vi "Example_OE1311&1351 Control.vi"() -> ()   [LabVIEW 2011]
uses:
  <vilib>/Utility/error.llb/DialogType.ctl
panel:
  out "loss count":i32=-1
  in  "Sample count":u32
  in  "buffer":u8
  out "Zero Data?":bool
  out "Queue out":errorcluster caption="error out"
  out "Queue output":refnum<queue>
  in  "Timeout":u32=100
  in  "Port":u32=10001
  in  "IP Address":string
  out "Freq":dbl
  out "xita":dbl
  out "R":dbl
  out "Input Overlaod":bool
  out "PLL Lock":bool
  out "Error":string
  out "Serial Versions":string
  in  "Table":T1(tab) caption="选项卡控件"
  in  "OE1300_Configure Input Filter":T2 {"Input Coupling" items=["AC", "DC"]; "Input Source" items=["A", "B", "Current"]}
  in  "OE1300_Configure Ref Phase":T3={"Reference Source"=0, "Internal Frequency(Hz)"=1000.0, "Phase  (degree)"=0.0, "External Ref Trigger"=0, "Instrument Mode "=4} {"Instrument Mode" items=["OE1311"=3, "OE1351"=4, "OE1301"=5]; "External Ref Trigger" items=["TTL Rising Edge", "TTL Fallling Edge", "Sine Zero Crossing"]; "Phase  (degree)" min=-180.0 max=180.0 format="%#.2g"; "Internal Frequency(Hz)" min=0.001 max=1002000.0 format="%#.3f"; "Reference Source" items=["External", "Internal", "Self"]}
  in  "OE1300_Configure Sens and Filter":T4={"Time Constant(s) "=0.1, "Low Pass Filter Slope "=1, "Enable Sync Filter "=0, "Input Range"=2} {"Input Range" items=["5 V/uA", "2 V/uA", "1 V/uA", "500 mV/nA", "200 mV/nA", "100 mV/nA", "50 mV/nA", "20 mV/nA", "10 mV/nA", "5 mV/nA", "2 mV/nA", "1 mV/nA", "500 uV/pA", "200 uV/pA", "100 uV/pA", "50 uV/pA", "20 uV/pA", "10 uV/pA", "5 uV/pA", "2 uV/pA", "1 uV/pA", "500 nV/fA", "200 nV/fA", "100 nV/fA", "50 nV/fA", "20 nV/fA", "10 nV/fA", "5 nV/fA", "2 nV/fA", "1 nV/fA"]; "Enable Sync Filter" items=["OFF", "ON"]; "Low Pass Filter Slope" items=["6 dB/oct", "12 dB/oct", "18 db/oct", "24 dB/oct", "30 dB/oct", "36 dB/oct", "42 dB/oct", "48 dB/oct"]; "Time Constant(s)" min=1e-06 max=3000.0}
  in  "OE1300_Configure Channel Out":T5={"CH2 Offset"=0.0, "CH1 Offset"=0.0, "CH2 Expand"=1, "CH1 Expand"=1, "AUX OUT1"=1.0, "AUX OUT2"=1.0, "CH 1"=3, "CH 2"=3} {"CH 2" items=["Fixed", "X", "Y", "R", "Theta", "Xh1", "Yh1", "Rh1", "Theta h1", "Xh2", "Yh2", "Rh2", "Theta h2", "Xh3", "Yh3", "Rh3", "Theta h3", "Rh4", "Xh4", "Yh4", "Theta h4", "Rh5", "Xh5", "Yh5", "Theta h5", "Rh6", "Xh6", "Yh6", "Theta h6", "Rh7", "Xh6", "Yh6", "Theta h7", "X_Noise", "Y_Noise", "Freq", "AuxIn1", "AuxIn2"]; "CH 1" items=["Fixed", "X", "Y", "R", "Theta", "Xh1", "Yh1", "Rh1", "Theta h1", "Xh2", "Yh2", "Rh2", "Theta h2", "Xh3", "Yh3", "Rh3", "Theta h3", "Rh4", "Xh4", "Yh4", "Theta h4", "Rh5", "Xh5", "Yh5", "Theta h5", "Rh6", "Xh6", "Yh6", "Theta h6", "Rh7", "Xh6", "Yh6", "Theta h7", "X_Noise", "Y_Noise", "Freq", "AuxIn1", "AuxIn2"]; "AUX OUT2" min=-10.0 max=10.0 format="%#.3g"; "AUX OUT1" min=-10.0 max=10.0 format="%#.3g"; "CH1 Expand" min=1 max=256; "CH2 Expand" min=1 max=256; "CH1 Offset" min=-100.0 max=100.0 format="%#.2g"; "CH2 Offset" min=-100.0 max=100.0 format="%#.2g"}
  in  "OE1300_Configure Sine Out":T6={"Sine Output Amplitude (V)"=0.1, "SineOut Mode"=0} {"SineOut Mode" items=["OFF", "Fixed"]; "Sine Output Amplitude (V)" min=0.0001 max=5.0 format="%#.4g"}
  in  "OE1300_Configure Demodulator":T7={"Demodulator"=1, "Mode"=0, "Arbitrary Frequency"=1000.0, "Harmonic"=1, "Instrument Mode "=4, "Phase  (degree)"=0.0} {"Phase  (degree)" min=-180.0 max=180.0 format="%#.2g"; "Instrument Mode" items=["OE1311"=3, "OE1351"=4, "OE1301"=5]; "Harmonic" min=1 max=32767; "Arbitrary Frequency" min=1e-06 max=1002000.0 format="%#.3f"; "Mode" items=["Harm", "Arb_Freq"]; "Demodulator" items=["1", "2", "3", "4", "5", "6", "7"]}
  in  "Save Button":bool
  in  "file path":path
  in  "Sample Rate":dbl=0.1 min=0.001 max=100.0
  out "Status":string
  in  "Connect":bool
  in  "VISA resource name":refnum<visa-resource-name>
  in  "Remote Mode":u16(ring)=1 items=["RS232"=1, "Ethernet"=3]
  in  "Baud Rate (115200)":u32=115200
  # "Tel          :   +86-020-84133345\nWebsite  :   www.ssi-instrument.com\nE-mail     :   support@si-instrument.com"
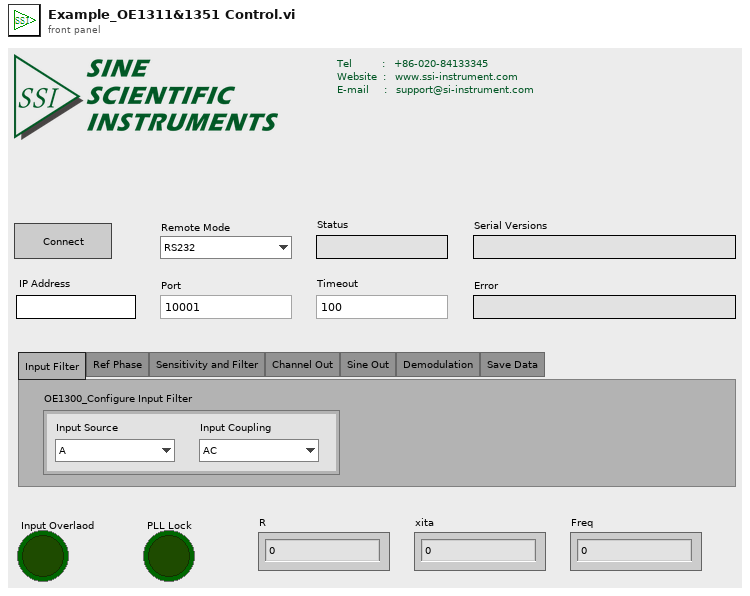
[diagram p1: front panel]
types:
  T1 = enum32{"Input Filter", "Ref Phase", "Sensitivity and Filter", "Channel Out", "Sine Out", "Demodulation", "Save Data"}
  T2 = cluster{"Input Source":u16, "Input Coupling ":u16}
  T3 = cluster{"Reference Source":u16, "Internal Frequency(Hz)":dbl, "Phase  (degree)":dbl, "External Ref Trigger":u16, "Instrument Mode ":u16}
  T4 = cluster{"Time Constant(s) ":dbl, "Low Pass Filter Slope ":u8, "Enable Sync Filter ":u16, "Input Range":u16}
  T5 = cluster{"CH2 Offset":dbl, "CH1 Offset":dbl, "CH2 Expand":i16, "CH1 Expand":i16, "AUX OUT1":dbl, "AUX OUT2":dbl, "CH 1":u16, "CH 2":u16}
  T6 = cluster{"Sine Output Amplitude (V)":dbl, "SineOut Mode":u8}
  T7 = cluster{"Demodulator":u16, "Mode":u16, "Arbitrary Frequency":dbl, "Harmonic":u16, "Instrument Mode ":u16, "Phase  (degree)":dbl}
  T8 = enum16{"OE1022", "OE1022D", "OE1201", "OE2031&OE2041", "OE1311&OE1351"}
  T9 = cluster{"Port":u32, "Timeout":u32, "IP Address":string}
  T10 = cluster{"PLL Lock(1: External Lock)":bool, "Input Overlaod":bool}
  T11 = cluster{"X":dbl, "Y":dbl, "R":dbl, "θ":dbl, "XD1":dbl, "YD1":dbl, "RD1":dbl, "θD1":dbl, "XD2":dbl, "YD2":dbl, "RD2":dbl, "θD2":dbl, "XD3":dbl, "YD3":dbl, "RD3":dbl, "θD3":dbl, "XD4":dbl, "YD4":dbl, "RD4":dbl, "θD4":dbl, "XD5":dbl, "YD5":dbl, "RD5":dbl, "θD5":dbl, "XD6":dbl, "YD6":dbl, "RD6":dbl, "θD6":dbl, "XD7":dbl, "YD7":dbl, "RD7":dbl, "θD7":dbl, "X-Noise":dbl, "Y-Noise":dbl, "Frequency":dbl, "AUX-IN1":dbl, "AUX-IN2":dbl}
  T12 = typedef "DialogType.ctl" = u16
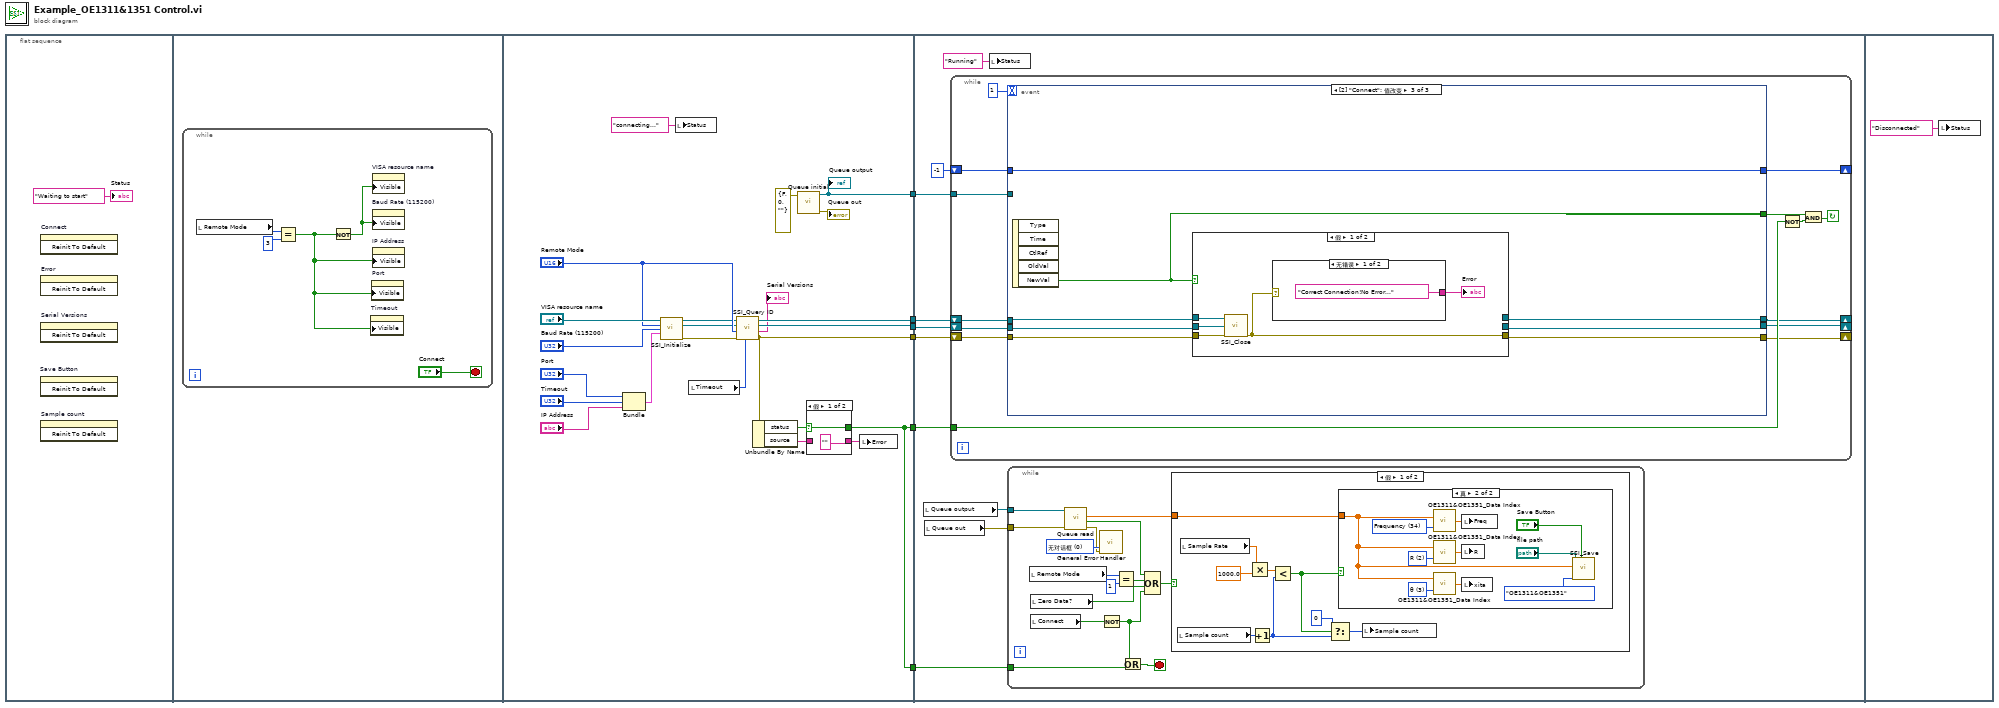
[diagram p0: block diagram]
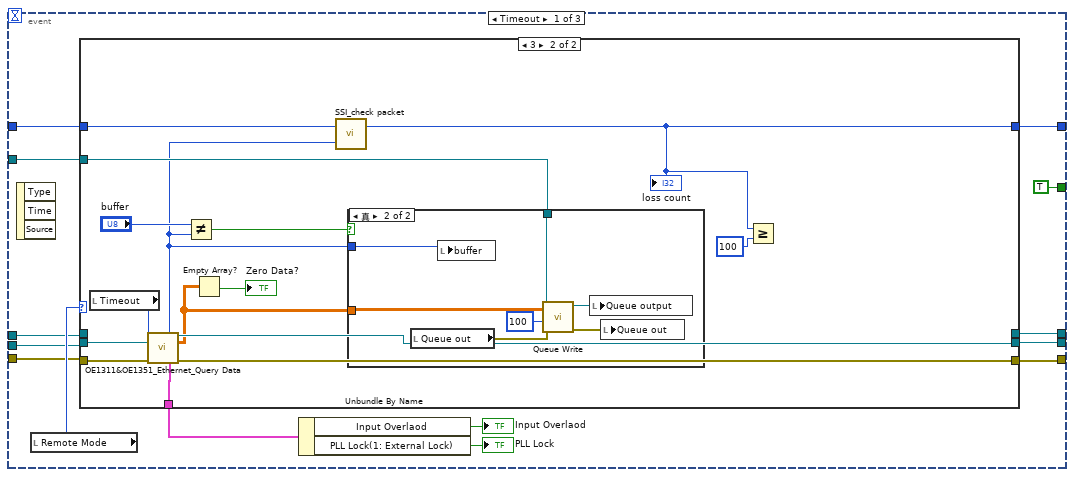
[diagram p5: hidden frame]
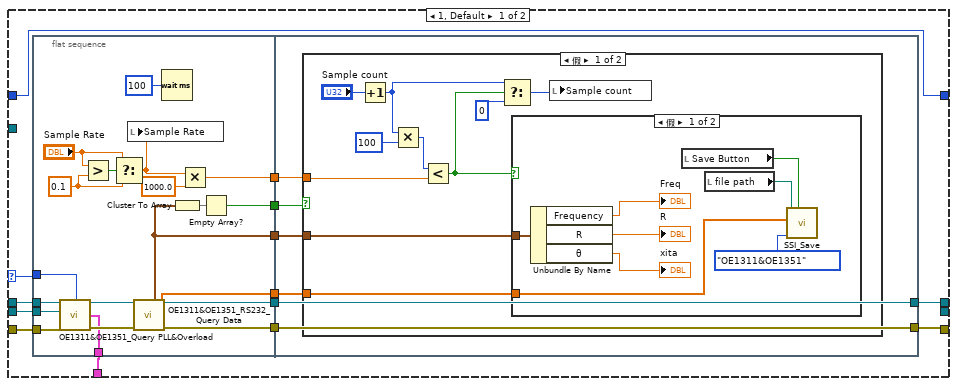
[diagram p6: hidden frame]
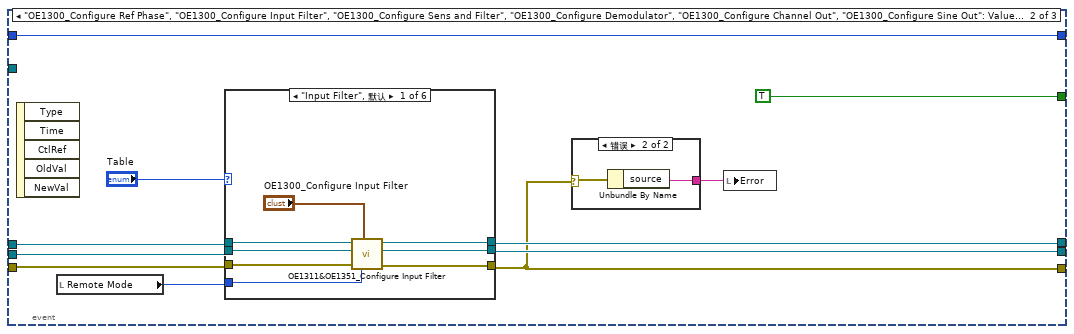
[diagram p10: hidden frame]
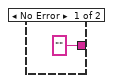
[diagram p11: hidden frame]
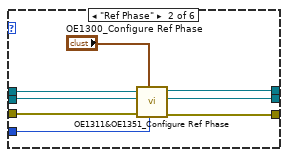
[diagram p12: hidden frame]
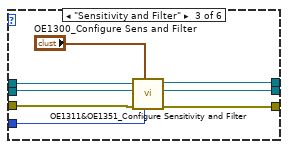
[diagram p13: hidden frame]
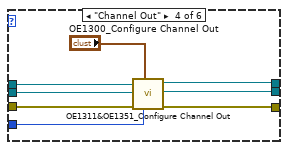
[diagram p14: hidden frame]
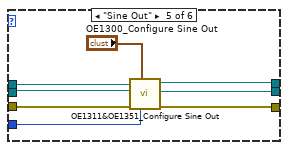
[diagram p15: hidden frame]
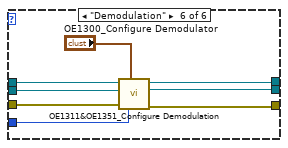
[diagram p16: hidden frame]
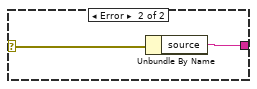
[diagram p17: hidden frame]
diagram:
  n1 = flat-sequence {
    tunnel: [w32] -> w6
    tunnel: [w31] -> w5
    tunnel: [w28] -> w4
    tunnel: [w16] -> w3
    tunnel: [w18] -> w2
    tunnel: [w16] -> w1
    tunnel: w6 -> [w48]
    tunnel: w5 -> [w47]
    tunnel: w4 -> [w46]
    tunnel: w3 -> [w45]
    tunnel: w2 -> [w42]
    tunnel: w1 -> [w40]
    frame #0 {
      n2 = invoke on="Save Button" class="Bool (严格)" method="Reinit To Default"() -> ()  [unwired: 3 in, 3 out]
      n3 = invoke on="Connect" class="Bool (严格)" method="Reinit To Default"() -> ()  [unwired: 3 in, 3 out]
      n4 = invoke on="Error" class="Str" method="Reinit To Default"() -> ()  [unwired: 3 in, 3 out]
      n5 = invoke on="Serial Versions" class="Str" method="Reinit To Default"() -> ()  [unwired: 3 in, 3 out]
      n6 = invoke on="Sample count" class="DigNum (严格)" method="Reinit To Default"() -> ()  [unwired: 3 in, 3 out]
      "Status" <- "Waiting to start" ("status")
    }
    frame #1 {
      n7 = while {
        stop <- "Connect" stop-if-true
        n8 = local read "Remote Mode"() -> (w10:u16)
        n9 = Equal?(x=w10, y=u16 3) -> (x = y?=w11:bool)
        n10 = Not(x=w11) -> (.not. x?=w8:bool)
        n11 = property on="Timeout" class="DigNum (严格)"("Visible"=w11) -> ()  [unwired: 2 in, 2 out]
        n12 = property on="Port" class="DigNum (严格)"("Visible"=w11) -> ()  [unwired: 2 in, 2 out]
        n13 = property on="VISA resource name" class="VISAName"("Visible"=w8) -> ()  [unwired: 2 in, 2 out]
        n14 = property on="Baud Rate (115200)" class="DigNum (严格)"("Visible"=w8) -> ()  [unwired: 2 in, 2 out]
        n15 = property on="IP Address" class="Str"("Visible"=w11) -> ()  [unwired: 2 in, 2 out]
      }
    }
    frame #2 {
      n16 = Bundle("Port"="Port", "Timeout"="Timeout", "IP Address"="IP Address") -> (w23:T9)  [unwired: 1 in]
      n17 = call "SSI_Initialize.vi"("VISA resource name"="VISA resource name", "Remote Mode"="Remote Mode", "baud rate (921600)"="Baud Rate (115200)", "Ethernet"=w23) -> ("VISA resource name out"=w13:refnum<visa-resource-name>, "connection ID(Ethernet)"=w14:refnum<k5>, "error out"=w15:errorcluster)  [unwired: 9 in]
      n18 = local write "Status"("connecting..." ("status")) -> ()
      n19 = local read "Timeout"() -> (w21:u32)
      n20 = call "SSI_Query ID.vi"("Timeout"=w21, "Error in (no error)"=w15, "Remote Mode"="Remote Mode", "Connection ID in"=w14, "VISA resource name"=w13) -> ("Error out"=w28:errorcluster, "Read Buffer"=→"Serial Versions":string, "Connection ID out"=w31:refnum<k5>, "VISA resource  out"=w32:refnum<visa-resource-name>)  [unwired: 3 in]
      n21 = Unbundle By Name(w28) -> ("status"=w29:bool, "source"=w27:string)
      n22 = call "Queue initial.vi"("Error in (no error)"=errorcluster {"status"=FALSE, "code"=0, "source"=""}) -> ("Error out"=→"Queue out":errorcluster, "Queue output"=w18:refnum<queue>)  [unwired: 9 in]
      "Queue output" <- w18
      n23 = case shown="假" w29 {
        selector: w29 -> [w37 w39]
        tunnel: [w37 w39] -> w16
        tunnel: ["" w38] -> w26
        tunnel: w27 -> [_ w38]
        frame False {
        }
        frame True {
        }
      }
      n24 = local write "Error"(w26) -> ()
    }
    frame #3 {
      n25 = local read "Queue output"() -> (w44:refnum<queue>)
      n26 = local read "Queue out"() -> (w43:errorcluster)
      n27 = while {
        tunnel: w45 -> [w93]
        tunnel: w42 -> [w89]
        shift-right: [w86] -> _
        shift-left: w48 -> [w92]
        shift-right: [w87] -> _
        shift-left: w47 -> [w91]
        shift-right: [w88] -> _
        shift-left: w46 -> [w90]
        shift-right: [w84] -> _
        shift-left: -1 ("loss count") -> [w85]
        stop <- w94 continue-if-true
        n28 = event shown="[2] \"Connect\": 值改变" {
          selector: _ -> [_ _ _]
          dyn-events: _ -> [_ _ _]
          timeout: 1 -> [_ _ _]
          tunnel: [TRUE ("NewVal") TRUE ("Stop") w260] -> w95
          tunnel: [w111 w197 w261] -> w88
          tunnel: [w103 w201 w255] -> w86
          tunnel: [w110 w200 w256] -> w87
          tunnel: w92 -> [w107 w195 w257]
          tunnel: w91 -> [w105 w194 w258]
          tunnel: w90 -> [w106 w193 w259]
          tunnel: w89 -> [w108 _ _]
          tunnel: w85 -> [w102 w192 w254]
          tunnel: [w101 w192 w254] -> w84
          event Timeout {
            n29 = event-data() -> ()  [unwired: 1 in, 3 out]
            n30 = local read "Remote Mode"() -> (w109:u16)
            n31 = case shown="3" w109 {
              selector: w109 -> [w119 _]
              tunnel: [w121 w180] -> w111
              tunnel: [_ w183] -> w110
              tunnel: w106 -> [w125 w182]
              tunnel: w105 -> [w124 w181]
              tunnel: w107 -> [w123 _]
              tunnel: w108 -> [_ w177]
              tunnel: [w120 w174] -> w104
              tunnel: [w122 _] -> w103
              tunnel: w102 -> [w112 w173]
              tunnel: [w112 w171] -> w101
              frame 1, Default {
                n32 = flat-sequence {
                  tunnel: w119 -> [w134]
                  tunnel: [w133] -> w118
                  tunnel: [w132] -> w117
                  tunnel: [w131] -> w116
                  tunnel: [w130] -> w115
                  tunnel: [w129] -> w114
                  tunnel: [w128] -> w113
                  tunnel: [w127] -> w120
                  tunnel: w125 -> [w137]
                  tunnel: w124 -> [w136]
                  tunnel: w123 -> [w135]
                  tunnel: w118 -> [w150]
                  tunnel: w117 -> [w151]
                  tunnel: [w151] -> w122
                  tunnel: [w150] -> w121
                  tunnel: w116 -> [w149]
                  tunnel: w115 -> [w148]
                  tunnel: w114 -> [w147]
                  tunnel: w113 -> [w146]
                  frame #0 {
                    w143 = 0.1 ("y")
                    n33 = call "OE1311&OE1351_Query PLL&Overload.vi"("VISA resource name"=w135, "Connection ID in"=w136, "Remote Mode"=w134, "Error in (no error)"=w137) -> ("VISA resource  out"=w138:refnum<visa-resource-name>, "OE1300_Query PLL&Overload"=w127:T10, "Error out"=w139:errorcluster)  [unwired: 7 in, 2 out]
                    n34 = Greater?(x="Sample Rate", y=w143) -> (0:w141:bool)
                    n35 = Select(t="Sample Rate", s=w141, f=w143) -> (s? t:f=w140:dbl)
                    n36 = local write "Sample Rate"(w140) -> ()
                    n37 = call "OE1311&OE1351_RS232_Query Data.vi"("VISA resource name"=w138, "Error in (no error)"=w139) -> ("VISA resource  out"=w132:refnum<visa-resource-name>, "Data Array"=w128:dbl[], "Parameter Values"=w129:T11, "Error out"=w133:errorcluster)  [unwired: 9 in, 1 out]
                    n38 = Wait (ms)(milliseconds to wait=u32 100 ("等待时间（毫秒）")) -> ()  [unwired: 1 out]
                    n39 = Cluster To Array(cluster=w129) -> (array=w145:dbl[])
                    n40 = Multiply(x=w140, y=1000.0) -> (x*y=w130:dbl)
                    n41 = Empty Array?(array=w145) -> (empty?=w131:bool)
                  }
                  frame #1 {
                    n42 = case shown="假" w149 {
                      tunnel: w148 -> [w158 _]
                      tunnel: w147 -> [w157 _]
                      tunnel: w146 -> [w156 _]
                      frame False {
                        n43 = Increment(x="Sample count") -> (x+1=w153:u32)
                        n44 = Multiply(x=w153, y=u32 100) -> (x*y=w160:u32)
                        n45 = Less?(x=w160, y=w158) -> (x < y?=w154:bool)
                        n46 = Select(t=w153, s=w154, f=u32 0 ("Loop count variable")) -> (s? t:f=w155:u32)
                        n47 = case shown="假" w154 {
                          tunnel: w157 -> [w163 _]
                          tunnel: w156 -> [w162 _]
                          frame False {
                            n48 = Unbundle By Name(w163) -> ("Frequency"=→"Freq":dbl, "R"=→"R":dbl, "θ"=→"xita":dbl)
                            n49 = local read "Save Button"() -> (w166:bool)
                            n50 = local read "file path"() -> (w165:path)
                            n51 = call "SSI_Save.vi"("file path (dialog if empty)"=w165, "1D data"=w162, "Instrument Mode"=T8."OE1311&OE1351", "Save Button"=w166) -> ()  [unwired: 7 in]
                          }
                          frame True {
                          }
                        }
                        n52 = local write "Sample count"(w155) -> ()
                      }
                      frame True {
                      }
                    }
                  }
                }
              }
              frame 3 {
                n53 = local read "Timeout"() -> (w184:u32)
                n54 = call "OE1311&OE1351_Ethernet_Query Data.vi"("Connection ID in"=w181, "Timeout"=w184, "Error in (no error)"=w182) -> ("Buffer Count"=w172:u8, "Connection ID out"=w183:refnum<k5>, "Total Date Array"=w176:dbl[][], "PLL&Overload"=w174:T10, "Error out"=w180:errorcluster)  [unwired: 5 in, 3 out]
                n55 = Not Equal?(x="buffer", y=w172) -> (x != y?=w178:bool)
                n56 = Empty Array?(array=w176) -> (empty?=→"Zero Data?":bool)
                n57 = call "SSI_check packet.vi"("input"=w172, "input loss"=w173) -> ("loss count"=w171:i32)  [unwired: 1 out]
                "loss count" <- w171
                n58 = case shown="真" w178 {
                  tunnel: w177 -> [_ w190]
                  tunnel: w172 -> [_ w186]
                  tunnel: w176 -> [_ w185]
                  frame False {
                  }
                  frame True {
                    n59 = local read "Queue out"() -> (w187:errorcluster)
                    n60 = local write "buffer"(w186) -> ()
                    n61 = call "Queue Write.vi"("Error in (no error)"=w187, "Group Count"=100, "Input Array"=w185, "Queue Input"=w190) -> ("Error out"=w188:errorcluster, "Queue output"=w189:refnum<queue>)  [unwired: 6 in]
                    n62 = local write "Queue output"(w189) -> ()
                    n63 = local write "Queue out"(w188) -> ()
                  }
                }
                n64 = Greater Or Equal?(x=w171, y=100) -> ()  [unwired: 1 out]
              }
            }
            n65 = Unbundle By Name(w104) -> ("Input Overlaod"=→"Input Overlaod":bool, "PLL Lock(1: External Lock)"=→"PLL Lock":bool)
          }
          event "OE1300_Configure Ref Phase", "OE1300_Configure Input Filter", "OE1300_Configure Sens and Filter", "OE1300_Configure Demodulator", "OE1300_Configure Channel Out", "OE1300_Configure Sine Out": Value Change {
            n66 = event-data() -> ()  [unwired: 1 in, 5 out]
            n67 = local read "Remote Mode"() -> (w199:u16)
            n68 = case shown="\"Input Filter\", 默认" "Table" {
              tunnel: [w211 w220 w228 w234 w243 w252] -> w201
              tunnel: [w212 w219 w229 w236 w245 w251] -> w197
              tunnel: [w213 w218 w227 w235 w244 w250] -> w200
              tunnel: w199 -> [w210 w217 w225 w237 w241 w253]
              tunnel: w195 -> [w208 w216 w224 w232 w240 w248]
              tunnel: w194 -> [w206 w215 w223 w231 w239 w247]
              tunnel: w193 -> [w207 w214 w222 w230 w238 w246]
              frame "Input Filter", Default {
                n69 = call "OE1311&OE1351_Configure Input Filter.vi"("OE1300_Configure Input Filter"="OE1300_Configure Input Filter", "Error in (no error)"=w207, "Remote Mode"=w210, "Connection ID in"=w206, "VISA resource name"=w208) -> ("Error out"=w212:errorcluster, "Connection ID out"=w213:refnum<k5>, "VISA resource  out"=w211:refnum<visa-resource-name>)  [unwired: 3 in, 1 out]
              }
              frame "Ref Phase" {
                n70 = call "OE1311&OE1351_Configure Ref Phase.vi"("OE1300_Configure Ref Phase"="OE1300_Configure Ref Phase", "Error in (no error)"=w214, "Remote Mode"=w217, "Connection ID in"=w215, "VISA resource name"=w216) -> ("Error out"=w219:errorcluster, "Connection ID out"=w218:refnum<k5>, "VISA resource  out"=w220:refnum<visa-resource-name>)  [unwired: 3 in, 1 out]
              }
              frame "Sensitivity and Filter" {
                n71 = call "OE1311&OE1351_Configure Sensitivity and Filter.vi"("OE1300_Configure \nSens and Filter"="OE1300_Configure Sens and Filter", "Error in (no error)"=w222, "Remote Mode"=w225, "Connection ID in"=w223, "VISA resource name"=w224) -> ("Error out"=w229:errorcluster, "Connection ID out"=w227:refnum<k5>, "VISA resource  out"=w228:refnum<visa-resource-name>)  [unwired: 3 in, 1 out]
              }
              frame "Channel Out" {
                n72 = call "OE1311&OE1351_Configure Channel Out.vi"("OE1300_Configure Channel Out"="OE1300_Configure Channel Out", "Error in (no error)"=w230, "Remote Mode"=w237, "Connection ID in"=w231, "VISA resource name"=w232) -> ("Error out"=w236:errorcluster, "Connection ID out"=w235:refnum<k5>, "VISA resource  out"=w234:refnum<visa-resource-name>)  [unwired: 3 in, 1 out]
              }
              frame "Sine Out" {
                n73 = call "OE1311&OE1351_Configure Sine Out.vi"("OE1300_Configure Sine Out"="OE1300_Configure Sine Out", "Error in (no error)"=w238, "Remote Mode"=w241, "Connection ID in"=w239, "VISA resource name"=w240) -> ("Error out"=w245:errorcluster, "Connection ID out"=w244:refnum<k5>, "VISA resource  out"=w243:refnum<visa-resource-name>)  [unwired: 3 in, 1 out]
              }
              frame "Demodulation" {
                n74 = call "OE1311&OE1351_Configure Demodulation.vi"("OE1300_Configure Demodulator"="OE1300_Configure Demodulator", "Error in (no error)"=w246, "Remote Mode"=w253, "Connection ID in"=w247, "VISA resource name"=w248) -> ("Error out"=w251:errorcluster, "Connection ID out"=w250:refnum<k5>, "VISA resource  out"=w252:refnum<visa-resource-name>)  [unwired: 3 in, 1 out]
              }
            }
            n75 = case shown="错误" w197 {
              selector: w197 -> [_ w205]
              tunnel: ["" ("source") w204] -> w196
              frame No Error {
              }
              frame Error {
                n76 = Unbundle By Name(w205) -> ("source"=w204:string)
              }
            }
            n77 = local write "Error"(w196) -> ()
          }
          event "Connect": Value Change {
            n78 = event-data() -> ("NewVal"=w260:bool)  [unwired: 1 in, 4 out]
            n79 = case shown="假" w260 {
              tunnel: [w266 w272] -> w261
              tunnel: w259 -> [w264 w272]
              tunnel: w258 -> [w263 w271]
              tunnel: w257 -> [w262 w270]
              tunnel: [_ w271] -> w256
              tunnel: [_ w270] -> w255
              frame False {
                n80 = call "SSI_Close.vi"("Error in (no error)"=w264, "Connection ID in"=w263, "VISA resource name"=w262) -> ("Error out"=w266:errorcluster)  [unwired: 4 in]
                n81 = case shown="无错误" w266 {
                  selector: w266 -> [_ w269]
                  tunnel: ["Correct Connection!No Error..." ("source") w268] -> w265
                  frame No Error {
                  }
                  frame Error {
                    n82 = Unbundle By Name(w269) -> ("source"=w268:string)
                  }
                }
                "Error" <- w265
              }
              frame True {
              }
            }
          }
        }
        n83 = Not(x=w93) -> (.not. x?=w96:bool)
        n84 = And(x=w95, y=w96) -> (x .and. y?=w94:bool)
      }
      n85 = local write "Status"("Running" ("status")) -> ()
      n86 = while {
        tunnel: w44 -> [w57]
        tunnel: w43 -> [w56]
        tunnel: w40 -> [w52]
        stop <- w50 stop-if-true
        w59 = T12 0 items=["无对话框", "确定信息", "继续或停止信息", "确定信息＋警告", "继续/停止+警告"] ("type of dialog (OK msg:1)")
        n87 = local read "Remote Mode"() -> (w64:u16)
        n88 = local read "Zero Data?"() -> (w60:bool)
        n89 = local read "Connect"() -> (w55:bool)
        n90 = call "Queue read.vi"("Error in (no error)"=w56, "Queue Input"=w57) -> ("Error out"=w58:errorcluster, "Timeout？"=w53:bool, "Output Array"=w54:sgl[])  [unwired: 7 in]
        n91 = call <vilib>:"General Error Handler.vi"("type of dialog (OK msg:1)"=w59, "error in (no error)"=w58) -> ()  [unwired: 9 in, 5 out]
        n92 = Not(x=w55) -> (.not. x?=w51:bool)
        n93 = Equal?(x=w64, y=u16 1) -> (x = y?=w61:bool)
        n94 = Or(x=w51, y=w52) -> (x .or. y?=w50:bool)
        n95 = Compound Arithmetic op=OR(w53, w61, w60, w51) -> (w62:bool)
        n96 = case shown="假" w62 {
          tunnel: w54 -> [w73 _]
          frame False {
            n97 = local read "Sample count"() -> (w70:u32)
            n98 = local read "Sample Rate"() -> (w72:dbl)
            n99 = Multiply(x=w72, y=1000.0) -> (x*y=w69:dbl)
            n100 = Increment(x=w70) -> (x+1=w65:u32)
            n101 = Less?(x=w69, y=w65) -> (x < y?=w68:bool)
            n102 = Select(t=u32 0 ("Loop count variable"), s=w68, f=w65) -> (s? t:f=w67:u32)
            n103 = case shown="真" w68 {
              tunnel: w73 -> [_ w79]
              frame False {
              }
              frame True {
                w74 = u16 3 items=["X", "Y", "R", "θ", "XD1", "YD1", "RD1", "θD1", "XD2", "YD2", "RD2", "θD2", "XD3", "YD3", "RD3", "θD3", "XD4", "YD4", "RD4", "θD4", "XD5", "YD5", "RD5", "θD5", "XD6", "YD6", "RD6", "θD6", "XD7", "YD7", "RD7", "θD7", "X_Noise", "Y_Noise", "Frequency", "AUX-IN1", "AUX-IN2"] ("Parameter Type")
                w75 = u16 2 items=["X", "Y", "R", "θ", "XD1", "YD1", "RD1", "θD1", "XD2", "YD2", "RD2", "θD2", "XD3", "YD3", "RD3", "θD3", "XD4", "YD4", "RD4", "θD4", "XD5", "YD5", "RD5", "θD5", "XD6", "YD6", "RD6", "θD6", "XD7", "YD7", "RD7", "θD7", "X_Noise", "Y_Noise", "Frequency", "AUX-IN1", "AUX-IN2"] ("Parameter Type")
                w76 = u16 34 items=["X", "Y", "R", "θ", "XD1", "YD1", "RD1", "θD1", "XD2", "YD2", "RD2", "θD2", "XD3", "YD3", "RD3", "θD3", "XD4", "YD4", "RD4", "θD4", "XD5", "YD5", "RD5", "θD5", "XD6", "YD6", "RD6", "θD6", "XD7", "YD7", "RD7", "θD7", "X_Noise", "Y_Noise", "Frequency", "AUX-IN1", "AUX-IN2"] ("Parameter Type")
                n104 = call "OE1311&OE1351_Data Index.vi"("Parameter Type"=w76, "Input Date Array"=w79) -> ("Parameter"=w80:dbl)
                n105 = call "OE1311&OE1351_Data Index.vi"("Parameter Type"=w75, "Input Date Array"=w79) -> ("Parameter"=w78:dbl)
                n106 = call "OE1311&OE1351_Data Index.vi"("Parameter Type"=w74, "Input Date Array"=w79) -> ("Parameter"=w77:dbl)
                n107 = local write "Freq"(w80) -> ()
                n108 = local write "R"(w78) -> ()
                n109 = local write "xita"(w77) -> ()
                n110 = call "SSI_Save.vi"("file path (dialog if empty)"="file path", "1D data"=w79, "Instrument Mode"=T8."OE1311&OE1351", "Save Button"="Save Button") -> ()  [unwired: 7 in]
              }
            }
            n111 = local write "Sample count"(w67) -> ()
          }
          frame True {
          }
        }
      }
    }
    frame #4 {
      n112 = local write "Status"("Disconnected" ("status")) -> ()
    }
  }
